vi "oa_Check Tach Pulses Data for Waveform Reference.vi"(7 "reset? (True)":bool=TRUE, 8 "error in (no error)":errorcluster, 9 "interpolated pulse positions":dbl[](array[numeric]) format="%.2f", 10 "speed profile":T1 {"speed [RPM]" format="%.2f"; "time [s]" format="%.2f"}, 11 "resampled signal":cluster{"r0":dbl, "dr":dbl, "Y":dbl[]}={"r0"=0.0, "dr"=1.0, "Y"=[]} {"r0" format="%.2p"; "dr" format="%.2p"; "Y" format="%.2f"}) -> (0 "error out":errorcluster, 1 "interpolated pulse positions out":dbl[](array[numeric]) format="%.2f", 2 "speed profile out":T1 {"speed [RPM]" format="%.2f"; "time [s]" format="%.2f"}, 3 "resampled signal out":cluster{"r0":dbl, "dr":dbl, "Y":dbl[]}={"r0"=0.0, "dr"=1.0, "Y"=[]} {"r0" format="%.2p"; "dr" format="%.2p"; "Y" format="%.2f"}, 5 "reset":bool)   [LabVIEW 2017]
uses:
  <vilib>/addons/Sound and Vibration/Order Analysis/Tach Process/SubVIs/speed profile.ctl
  <vilib>/addons/Sound and Vibration/Order Analysis/Tach Process/SoundVib_TachProcess.lvlib
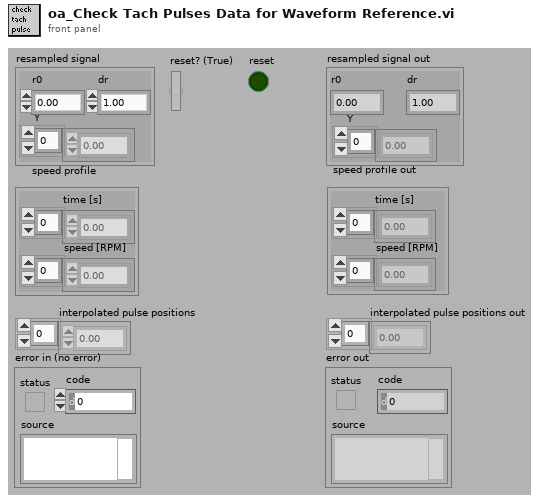
[diagram p1: front panel]
types:
  T1 = typedef "SoundVib_TachProcess.lvlib/speed profile.ctl" = cluster{"time [s]":dbl[], "speed [RPM]":dbl[]}
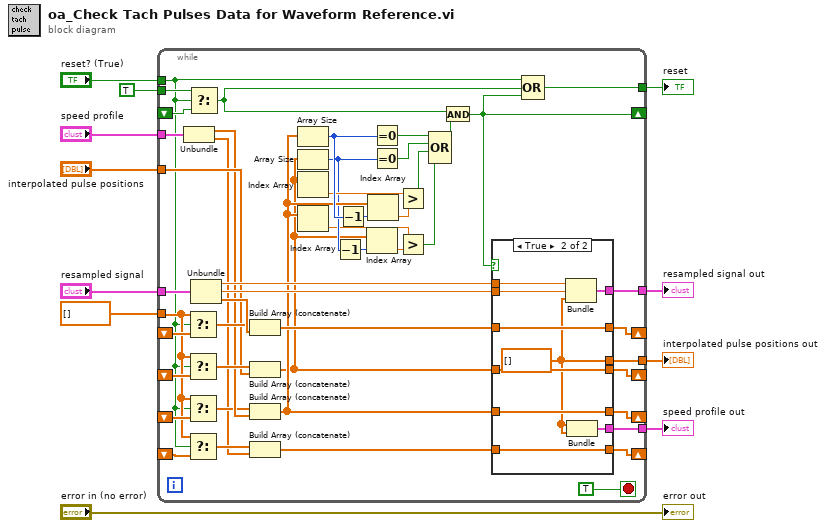
[diagram p0: block diagram]
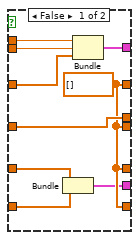
[diagram p2: hidden frame]
diagram:
  n1 = while {
    tunnel: "reset? (True)" -> [w30]
    shift-right: [w12] -> _
    shift-left: _ -> [w58]
    tunnel: "interpolated pulse positions" -> [w45]
    tunnel: "speed profile" -> [w57]
    tunnel: "resampled signal" -> [w55]
    shift-right: [w52] -> _
    shift-left: _ -> [w56]
    tunnel: dbl[] [] ("Y") -> [w37]
    tunnel: [w49] -> w5
    shift-right: [w44] -> _
    shift-left: _ -> [w47]
    tunnel: [w43] -> w4
    shift-right: [w40] -> _
    shift-left: _ -> [w42]
    shift-right: [w34] -> _
    shift-left: _ -> [w36]
    tunnel: [w32] -> w3
    tunnel: TRUE -> [w31]
    tunnel: [w13] -> w1
    stop <- TRUE stop-if-true
    n2 = Unbundle(w57) -> ("time [s]"=w41:dbl[], "speed [RPM]"=w35:dbl[])
    n3 = Select(t=w37, s=w30, f=w56) -> (s? t:f=w48:dbl[])
    n4 = Select(t=w37, s=w30, f=w47) -> (s? t:f=w46:dbl[])
    n5 = Select(t=w37, s=w30, f=w42) -> (s? t:f=w38:dbl[])
    n6 = Select(t=w37, s=w30, f=w36) -> (s? t:f=w39:dbl[])
    n7 = Select(t=w31, s=w30, f=w58) -> (s? t:f=w15:bool)
    n8 = Unbundle(w55) -> ("r0"=w50:dbl, "dr"=w51:dbl, "Y"=w54:dbl[])
    n9 = Build Array (concatenate)(w48, w54) -> (w53:dbl[])
    n10 = Build Array (concatenate)(w46, w45) -> (w23:dbl[])
    n11 = Build Array (concatenate)(w38, w41) -> (w26:dbl[])
    n12 = Build Array (concatenate)(w39, w35) -> (w33:dbl[])
    n13 = Array Size(array=w26) -> (size(s)=w29:i32)
    n14 = Array Size(array=w23) -> (size(s)=w24:i32)
    n15 = Index Array(array=w23) -> (element=w28:dbl)  [unwired: 1 in]
    n16 = Index Array(array=w26) -> (element=w20:dbl)  [unwired: 1 in]
    n17 = Decrement(x=w24) -> (x-1=w22:i32)
    n18 = Decrement(x=w29) -> (x-1=w25:i32)
    n19 = Index Array(array=w23, index=w22) -> (element=w21:dbl)
    n20 = Index Array(array=w26, index=w25) -> (element=w27:dbl)
    n21 = Equal To 0?(x=w29) -> (x = 0?=w19:bool)
    n22 = Equal To 0?(x=w24) -> (x = 0?=w18:bool)
    n23 = Greater?(x=w28, y=w27) -> (0:w17:bool)
    n24 = Greater?(x=w20, y=w21) -> (0:w16:bool)
    n25 = Compound Arithmetic op=OR(w19, w18, w17, w16) -> (w14:bool)
    n26 = And(x=w15, y=w14) -> (x .and. y?=w12:bool)
    n27 = case shown="True" w12 {
      tunnel: w53 -> [w68 w77]
      tunnel: [w61 w77] -> w52
      tunnel: w51 -> [w67 w72]
      tunnel: w50 -> [w66 w73]
      tunnel: [w65 w71] -> w49
      tunnel: w23 -> [w64 w76]
      tunnel: [w61 w76] -> w44
      tunnel: [w64 w70] -> w43
      tunnel: w26 -> [w63 w75]
      tunnel: [w61 w75] -> w40
      tunnel: [w61 w74] -> w34
      tunnel: w33 -> [w62 w74]
      tunnel: [w60 w69] -> w32
      frame False {
        w61 = dbl[] []
        n28 = Bundle(w63, w62) -> (w60:cluster{dbl[], dbl[]})  [unwired: 1 in]
        n29 = Bundle("r0"=w66, "dr"=w67, w68) -> (w65:cluster{"r0":dbl, "dr":dbl, dbl[]})  [unwired: 1 in]
      }
      frame True {
        w70 = dbl[] []
        n30 = Bundle("r0"=w73, "dr"=w72, w70) -> (w71:cluster{"r0":dbl, "dr":dbl, dbl[]})  [unwired: 1 in]
        n31 = Bundle(w70, w70) -> (w69:cluster{dbl[], dbl[]})  [unwired: 1 in]
      }
    }
    n32 = Compound Arithmetic op=OR(w30, w15, w12) -> (w13:bool)
  }
  "interpolated pulse positions out" <- w4
  "speed profile out" <- w3
  "reset" <- w1
  "resampled signal out" <- w5
  "error out" <- "error in (no error)"
